vi "Refresh Auth.vi"(6 "Google":refnum<class "Google.lvclass">, 7 "Authorization in":refnum<class "Authorization.lvclass">, 8 "error in (no error)":errorcluster, 11 "Gmail in":refnum<class "Gmail.lvclass">) -> (0 "error out":errorcluster, 3 "Gmail out":refnum<class "Gmail.lvclass">, 5 "Authorization":refnum<class "Authorization.lvclass">)   [LabVIEW 2020, in "Gmail API.lvlib" / "Gmail.lvclass"]
uses:
  Gmail.lvclass
  <vilib>/IlluminatedG/IG OAuth2/OAuth2/Authorization/Authorization.lvclass
  <vilib>/IlluminatedG/IG OAuth2/OAuth2/Google/Google.lvclass
  C:/Program Files (x86)/National Instruments/LabVIEW 2020/vi.lib/IlluminatedG/IG OAuth2/OAuth2/OAuth2/OAuth2.lvclass
  <vilib>/IlluminatedG/IG OAuth2/OAuth2/OAuth2/OAuth2.lvclass
  <vilib>/IlluminatedG/IG OAuth2/OAuth2/Async Authorization/Async Authorization.lvclass
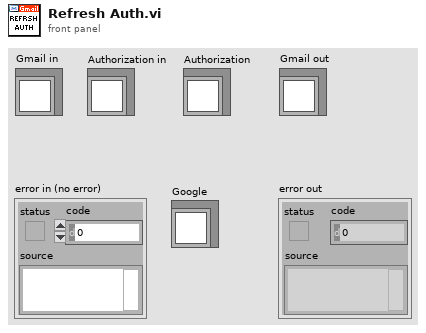
[diagram p1: front panel]
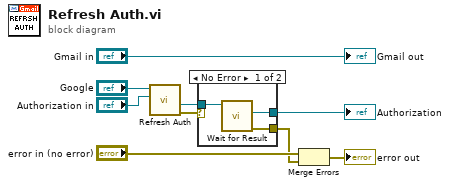
[diagram p0: block diagram]
diagram:
  n1 = call <vilib>:"Refresh Auth.vi"("Authorization in"="Authorization in", "OAuth2 in"="Google") -> ("error out"=w5:errorcluster, "Async Authentication"=w6:refnum<class "Async Authorization.lvclass">)  [unwired: 7 in, 1 out]
  n2 = case shown="No Error" w5 {
    selector: w5 -> [_ w13]
    tunnel: w6 -> [w12 _]
    tunnel: [w11 w13] -> w2
    tunnel: [w10 _] -> w4
    frame No Error {
      n3 = call <vilib>:"Wait for Result.vi"("Async Authorization in"=w12) -> ("error out"=w11:errorcluster, "Authorization"=w10:refnum<class "Authorization.lvclass">)  [unwired: 8 in, 1 out]
    }
    frame Error {
    }
  }
  "Authorization" <- w4
  n4 = Merge Errors("error in (no error)", w2) -> (→"error out":errorcluster)
  "Gmail out" <- "Gmail in"
